vi "Lookup Module by Type.vi"(7 "Force Enumerate (F)":bool, 8 "error in (no error)":errorcluster, 10 "Module Type":string) -> (0 "error out":errorcluster, 2 "Module Type":refnum<class "Module.lvclass">)   [LabVIEW 2020, in "Volatus.lvlib" / "VolatusAPI.lvclass"]
uses:
  VolatusAPI.lvclass
  Module/Module.lvclass
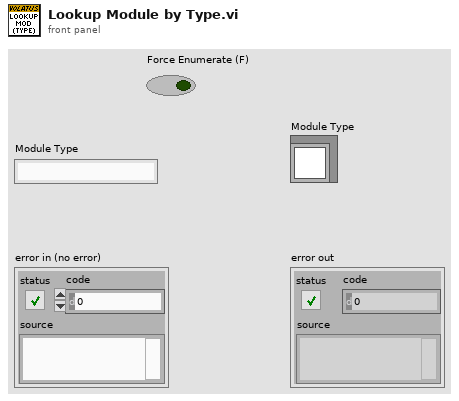
[diagram p1: front panel]
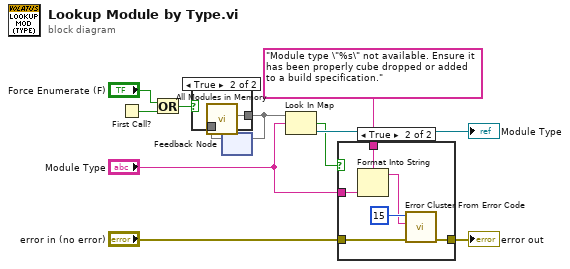
[diagram p0: block diagram]
diagram:
  n1 = First Call?() -> (First Call?: T/F=w11:bool)
  n2 = Or(x="Force Enumerate (F)", y=w11) -> (x .or. y?=w9:bool)
  n3 = feedback #1() -> (w8:map{string, refnum<class "Module.lvclass">})  [unwired: 1 in]
  n4 = case shown="True" w9 {
    tunnel: [w12 w13] -> w7
    tunnel: w8 -> [w12 _]
    frame False {
    }
    frame True {
      n5 = call "All Modules in Memory.vi"() -> ("Modules"=w13:map{string, refnum<class "Module.lvclass">})  [unwired: 11 in]
    }
  }
  n6 = feedback-in #1(w7) -> ()
  n7 = Look In Map(map=w7, key="Module Type") -> (key not found?=w1:bool, value=→"Module Type":refnum<class "Module.lvclass">)  [unwired: 1 in]
  n8 = case shown="True" w1 {
    tunnel: "error in (no error)" -> [w14 w20]
    tunnel: [w14 w19] -> w4
    tunnel: "Module type \"%s\" not available. Ensure it has been properly cube dropped or added to a build specification." -> [_ w17]
    tunnel: "Module Type" -> [_ w16]
    frame False {
    }
    frame True {
      n9 = Format Into String(format string=w17, w16) -> (resulting string=w15:string)  [unwired: 2 in, 1 out]
      n10 = call <vilib>:"Error Cluster From Error Code.vi"("error in (no error)"=w20, "error message (\"\")"=w15, "error code (0)"=15) -> ("error out"=w19:errorcluster)  [unwired: 6 in]
    }
  }
  "error out" <- w4
